vi "User Management.vi"() -> ()   [LabVIEW 2017]
uses:
  <vilib>/Utility/error.llb/DialogType.ctl
  Control/Login Authority CSV FGV Command.ctl
  Global/CHICTSO/Cikautxo Intermix Login Details.vi
panel:
  out "error out":errorcluster
  in  "error in (no error)":errorcluster
  in  "User data":T1
  in  "Delete":bool
  in  "New":bool
  in  "Exit":bool
  in  "Save":bool
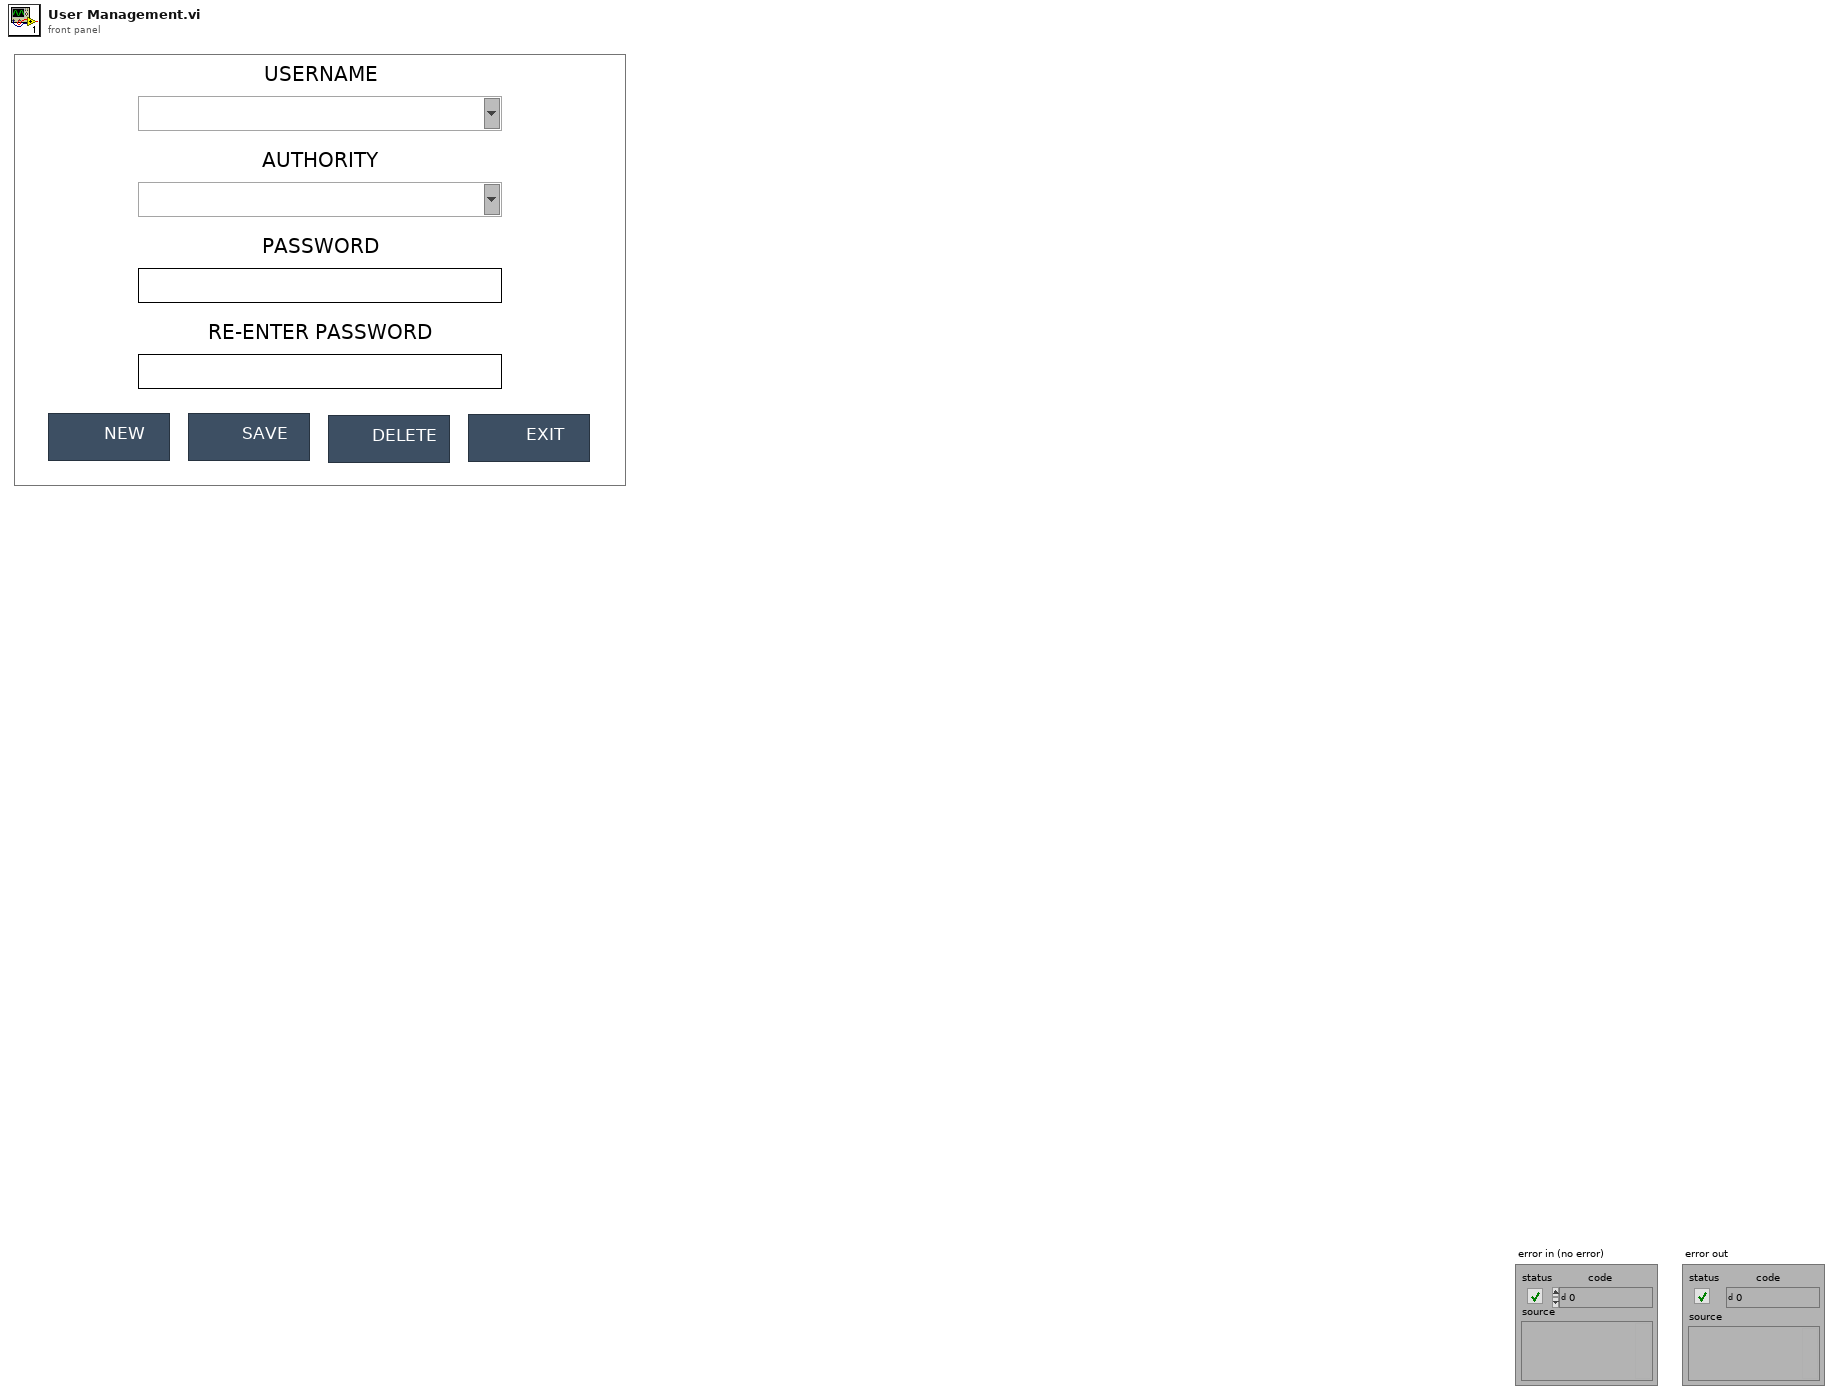
[diagram p1: front panel]
types:
  T1 = cluster{"USERNAME":string, "AUTHORITY":string, "PASSWORD":string, "RE-ENTER PASSWORD":string}
  T2 = typedef "Login Authority CSV FGV Command.ctl" = enum16{"Init", "Save", "Read", "Get Data", "Delete"}
  T3 = typedef "DialogType.ctl" = u16
  T4 = enum32{"invalid app kind", "Development System", "Run Time System", "Student Edition", "Embedded LabVIEW", "Evaluation", "Custom"}
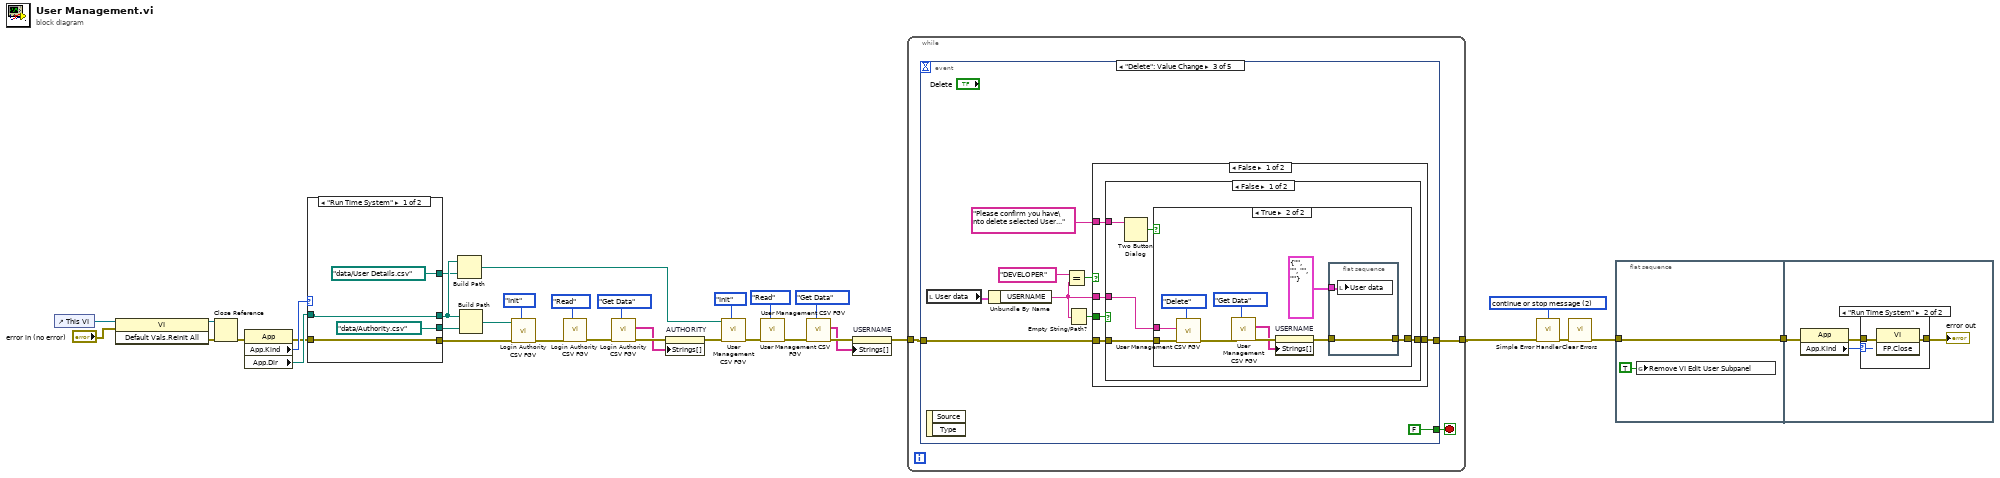
[diagram p0: block diagram]
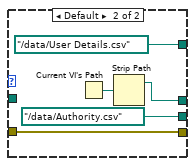
[diagram p3: hidden frame]
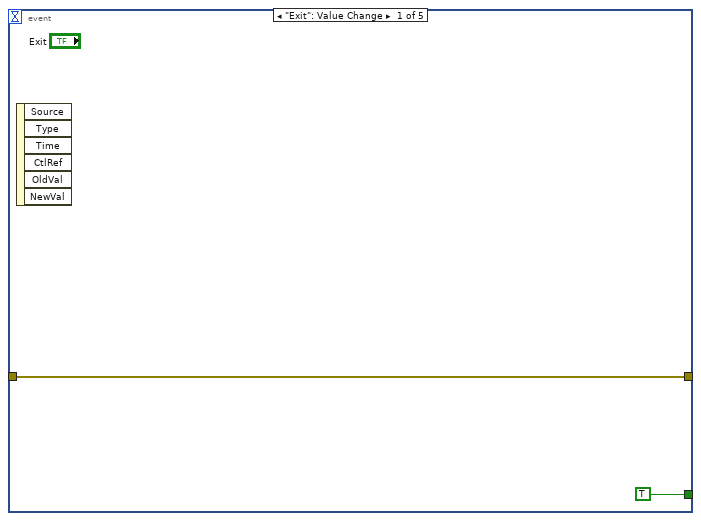
[diagram p4: hidden frame]
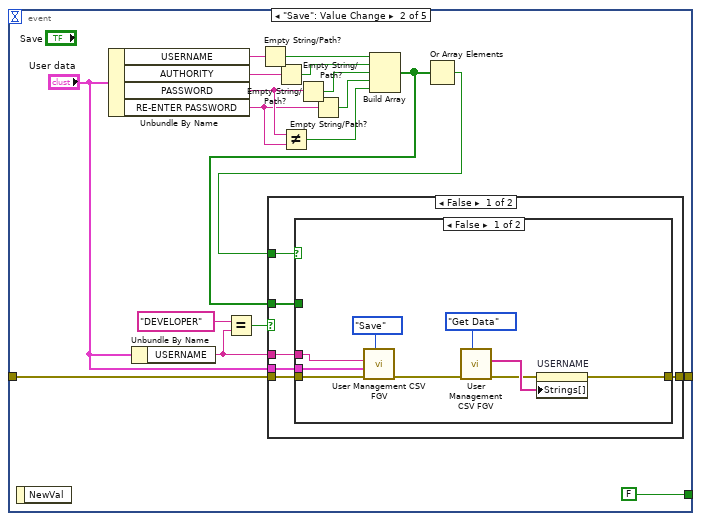
[diagram p5: hidden frame]
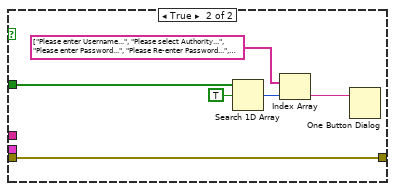
[diagram p6: hidden frame]
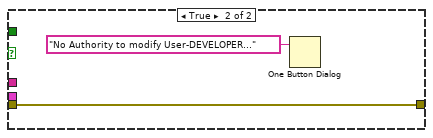
[diagram p7: hidden frame]
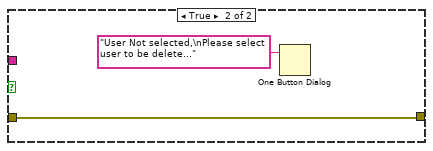
[diagram p9: hidden frame]
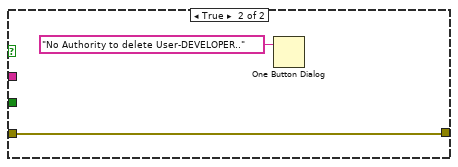
[diagram p10: hidden frame]
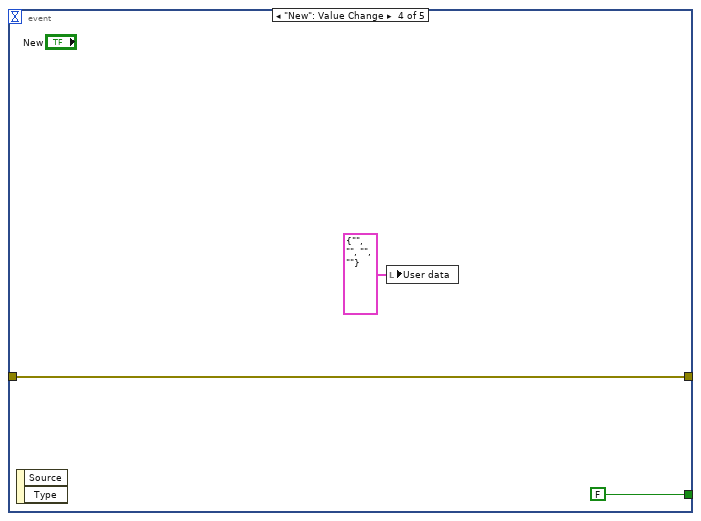
[diagram p11: hidden frame]
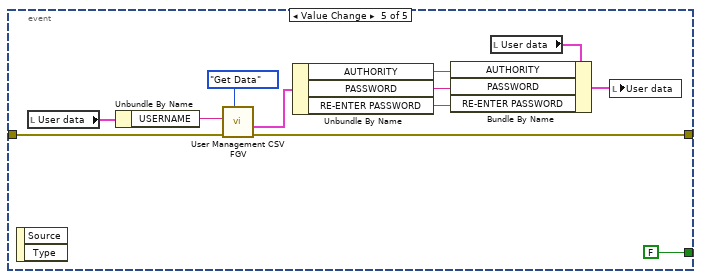
[diagram p12: hidden frame]
diagram:
  w15 = T3 2 items=["no dialog", "OK message", "continue or stop message", "OK message + warnings", "continue/stop + warnings"] ("type of dialog (OK msg:1)")
  n1 = control-ref of="This VI"() -> (w35:refnum<vi>)
  n2 = invoke class="VI" method="Default Vals.Reinit All"(reference=w35, error in="error in (no error)") -> (reference out=w32:refnum<vi>, error out=w33:errorcluster)  [unwired: 1 in, 1 out]
  n3 = Close Reference(reference=w32, error in (no error)=w33) -> (error out=w29:errorcluster)
  n4 = property class="App"(error in=w29) -> (error out=w28:errorcluster, "App.Kind"=w31:T4, "App.Dir"=w30:path)  [unwired: 1 in, 1 out]
  n5 = case shown="\"Run Time System\"" w31 {
    tunnel: w30 -> [w39 _]
    tunnel: [path "data/Authority.csv" ("path") path "../data/Authority.csv" ("path")] -> w27
    tunnel: [w39 w42] -> w13
    tunnel: w28 -> [w37 w41]
    tunnel: [w37 w41] -> w19
    tunnel: [path "data/User Details.csv" ("path") path "../data/User Details.csv" ("path")] -> w12
    frame "Run Time System" {
    }
    frame Default {
      n6 = Current VI's Path() -> (path=w43:path)
      n7 = Strip Path(path=w43) -> (stripped path=w42:path)  [unwired: 1 out]
    }
  }
  n8 = Build Path(base path=w13, name or relative path=w12) -> (appended path=w8:path)
  n9 = Build Path(base path=w13, name or relative path=w27) -> (appended path=w18:path)
  n10 = call "Login Authority CSV FGV.vi"("Command"=Login_Authority_CSV_FGV_Command."Init", "error in (no error)"=w19, "Path"=w18) -> ("error out"=w23:errorcluster)  [unwired: 6 in, 2 out]
  n11 = call "Login Authority CSV FGV.vi"("Command"=Login_Authority_CSV_FGV_Command."Read", "error in (no error)"=w23) -> ("error out"=w22:errorcluster)  [unwired: 7 in, 2 out]
  n12 = call "Login Authority CSV FGV.vi"("Command"=Login_Authority_CSV_FGV_Command."Get Data", "error in (no error)"=w22) -> ("error out"=w21:errorcluster, "Authorities"=w20:string[])  [unwired: 7 in, 1 out]
  n13 = property on="AUTHORITY" class="CmbBox"(error in=w21, "Strings[]"=w20) -> (error out=w9:errorcluster)  [unwired: 1 in, 1 out]
  n14 = call "User Management CSV FGV.vi"("Command"=Login_Authority_CSV_FGV_Command."Init", "error in (no error)"=w9, "Path"=w8) -> ("error out"=w11:errorcluster)  [unwired: 6 in, 2 out]
  n15 = call "User Management CSV FGV.vi"("Command"=Login_Authority_CSV_FGV_Command."Read", "error in (no error)"=w11) -> ("error out"=w10:errorcluster)  [unwired: 7 in, 2 out]
  n16 = call "User Management CSV FGV.vi"("Command"=Login_Authority_CSV_FGV_Command."Get Data", "error in (no error)"=w10) -> ("error out"=w4:errorcluster, "Usernames"=w2:string[])  [unwired: 7 in, 1 out]
  n17 = property on="USERNAME" class="CmbBox"(error in=w4, "Strings[]"=w2) -> (error out=w3:errorcluster)  [unwired: 1 in, 1 out]
  n18 = while {
    tunnel: w3 -> [w47]
    tunnel: [w46] -> w14
    stop <- w45 stop-if-true
    n19 = event shown="[2] \"Delete\": Value Change" {
      selector: _ -> [_ _ _ _ _]
      dyn-events: _ -> [_ _ _ _ _]
      timeout: _ -> [_ _ _ _ _]
      tunnel: w47 -> [w49 w56 w97 w128 w141]
      tunnel: [w49 w54 w96 w128 w140] -> w46
      tunnel: [TRUE FALSE FALSE FALSE FALSE] -> w45
      event "Exit": Value Change {
        n20 = event-data() -> ()  [unwired: 1 in, 6 out]
      }
      event "Save": Value Change {
        n21 = event-data() -> ()  [unwired: 1 in, 1 out]
        n22 = Unbundle By Name("User data") -> ("USERNAME"=w66:string, "AUTHORITY"=w65:string, "PASSWORD"=w60:string, "RE-ENTER PASSWORD"=w59:string)
        n23 = Unbundle By Name("User data") -> ("USERNAME"=w51:string)
        n24 = Equal?(x="DEVELOPER", y=w51) -> (x = y?=w50:bool)
        n25 = Empty String/Path?(string/path=w66) -> (empty?=w64:bool)
        n26 = Empty String/Path?(string/path=w65) -> (empty?=w63:bool)
        n27 = Not Equal?(x=w60, y=w59) -> (x != y?=w58:bool)
        n28 = Empty String/Path?(string/path=w60) -> (empty?=w62:bool)
        n29 = Empty String/Path?(string/path=w59) -> (empty?=w61:bool)
        n30 = Build Array(w64, w63, w62, w61, w58) -> (w53:bool[])
        n31 = Or Array Elements(Boolean array=w53) -> (logical OR=w57:bool)
        n32 = case shown="False" w50 {
          tunnel: w57 -> [w73 _]
          tunnel: w56 -> [w72 w90]
          tunnel: "User data" -> [w71 _]
          tunnel: w51 -> [w70 _]
          tunnel: [w69 w90] -> w54
          tunnel: w53 -> [w68 _]
          frame False {
            n33 = case shown="False" w73 {
              tunnel: w72 -> [w82 w88]
              tunnel: w71 -> [w80 _]
              tunnel: w70 -> [w79 _]
              tunnel: [w74 w88] -> w69
              tunnel: w68 -> [_ w87]
              frame False {
                n34 = call "User Management CSV FGV.vi"("Command"=Login_Authority_CSV_FGV_Command."Save", "error in (no error)"=w82, "User data In"=w80, "Username"=w79) -> ("error out"=w75:errorcluster)  [unwired: 5 in, 2 out]
                n35 = call "User Management CSV FGV.vi"("Command"=Login_Authority_CSV_FGV_Command."Get Data", "error in (no error)"=w75) -> ("error out"=w77:errorcluster, "Usernames"=w78:string[])  [unwired: 7 in, 1 out]
                n36 = property on="USERNAME" class="CmbBox"(error in=w77, "Strings[]"=w78) -> (error out=w74:errorcluster)  [unwired: 1 in, 1 out]
              }
              frame True {
                n37 = Search 1D Array(1D array=w87, element=TRUE) -> (index of element=w85:i32)  [unwired: 1 in]
                n38 = Index Array(array=string[] ["Please enter Username...", "Please select Authority...", "Please enter Password...", "Please Re-enter Password...", "Password & Re-entered Password\nare not matching..."], index=w85) -> (element=w84:string)
                n39 = One Button Dialog(message=w84) -> ()  [unwired: 1 in, 1 out]
              }
            }
          }
          frame True {
            n40 = One Button Dialog(message="No Authority to modify User-DEVELOPER...") -> ()  [unwired: 1 in, 1 out]
          }
        }
      }
      event "Delete": Value Change {
        n41 = local read "User data"() -> (w99:T1)
        n42 = event-data() -> ()  [unwired: 1 in, 2 out]
        n43 = Unbundle By Name(w99) -> ("USERNAME"=w93:string)
        n44 = Equal?(x="DEVELOPER", y=w93) -> (x = y?=w91:bool)
        n45 = Empty String/Path?(string/path=w93) -> (empty?=w95:bool)
        n46 = case shown="False" w91 {
          tunnel: w97 -> [w104 w126]
          tunnel: [w103 w126] -> w96
          tunnel: w95 -> [w102 _]
          tunnel: "Please confirm you have\nto delete selected User..." ("message") -> [w101 _]
          tunnel: w93 -> [w100 _]
          frame False {
            n47 = case shown="False" w102 {
              tunnel: w104 -> [w109 w123]
              tunnel: w100 -> [w108 _]
              tunnel: [w107 w123] -> w103
              tunnel: w101 -> [w105 _]
              frame False {
                n48 = Two Button Dialog(message=w105) -> (T button?=w106:bool)  [unwired: 2 in]
                n49 = case shown="True" w106 {
                  tunnel: w109 -> [w110 w119]
                  tunnel: w108 -> [_ w118]
                  tunnel: [w110 w112] -> w107
                  frame False {
                  }
                  frame True {
                    n50 = call "User Management CSV FGV.vi"("Command"=Login_Authority_CSV_FGV_Command."Delete", "error in (no error)"=w119, "Username"=w118) -> ("error out"=w116:errorcluster)  [unwired: 6 in, 2 out]
                    n51 = call "User Management CSV FGV.vi"("Command"=Login_Authority_CSV_FGV_Command."Get Data", "error in (no error)"=w116) -> ("error out"=w115:errorcluster, "Usernames"=w114:string[])  [unwired: 7 in, 1 out]
                    n52 = property on="USERNAME" class="CmbBox"(error in=w115, "Strings[]"=w114) -> (error out=w113:errorcluster)  [unwired: 1 in, 1 out]
                    n53 = flat-sequence {
                      tunnel: w113 -> [w122]
                      tunnel: [w122] -> w112
                      tunnel: T1 {"USERNAME"="", "AUTHORITY"="", "PASSWORD"="", "RE-ENTER PASSWORD"=""} ("User data") -> [w121]
                      frame #0 {
                        n54 = local write "User data"(w121) -> ()
                      }
                    }
                  }
                }
              }
              frame True {
                n55 = One Button Dialog(message="User Not selected,\nPlease select user to be delete...") -> ()  [unwired: 1 in, 1 out]
              }
            }
          }
          frame True {
            n56 = One Button Dialog(message="No Authority to delete User-DEVELOPER..") -> ()  [unwired: 1 in, 1 out]
          }
        }
      }
      event "New": Value Change {
        n57 = event-data() -> ()  [unwired: 1 in, 2 out]
        n58 = local write "User data"(T1 {"USERNAME"="", "AUTHORITY"="", "PASSWORD"="", "RE-ENTER PASSWORD"=""} ("User data")) -> ()
      }
      event "User data.USERNAME": Value Change {
        n59 = event-data() -> ()  [unwired: 1 in, 2 out]
        n60 = local read "User data"() -> (w138:T1)
        n61 = Unbundle By Name(w138) -> ("USERNAME"=w137:string)
        n62 = call "User Management CSV FGV.vi"("Command"=Login_Authority_CSV_FGV_Command."Get Data", "error in (no error)"=w141, "Username"=w137) -> ("error out"=w140:errorcluster, "User data Out"=w135:T1)  [unwired: 6 in, 1 out]
        n63 = Unbundle By Name(w135) -> ("AUTHORITY"=w133:string, "PASSWORD"=w132:string, "RE-ENTER PASSWORD"=w131:string)
        n64 = local read "User data"() -> (w134:T1)
        n65 = Bundle By Name(cluster=w134, "AUTHORITY"=w133, "PASSWORD"=w132, "RE-ENTER PASSWORD"=w131) -> (w130:T1)
        n66 = local write "User data"(w130) -> ()
      }
    }
  }
  n67 = call <vilib>:"Simple Error Handler.vi"("type of dialog (OK msg:1)"=w15, "error in (no error)"=w14) -> ("error out"=w17:errorcluster)  [unwired: 3 in, 4 out]
  n68 = call <vilib>:"Clear Errors.vi"("error in (no error)"=w17) -> ("error out"=w16:errorcluster)  [unwired: 5 in, 1 out]
  n69 = flat-sequence {
    tunnel: w16 -> [w143]
    tunnel: [w143] -> w1
    tunnel: w1 -> [w145]
    frame #0 {
      n70 = global write "Cikautxo Intermix Login Details.vi" "Remove VI Edit User Subpanel"(TRUE ("Remove VI Edit User Subpanel")) -> ()
    }
    frame #1 {
      n71 = property class="App"(error in=w145) -> (error out=w146:errorcluster, "App.Kind"=w147:T4)  [unwired: 1 in, 1 out]
      n72 = case shown="\"Run Time System\"" w147 {
        tunnel: w146 -> [w148 w150]
        tunnel: [w148 w149] -> w144
        frame Default {
        }
        frame "Run Time System" {
          n73 = invoke class="VI" method="FP.Close"(error in=w150) -> (error out=w149:errorcluster)  [unwired: 2 in, 2 out]
        }
      }
      "error out" <- w144
    }
  }
